vi "SV Read All Data.vi"(7 "reader ID":string="AllData", 8 "error in (no error)":errorcluster, 11 "buffer":refnum<data-value>) -> (0 "error out":errorcluster, 2 "waveforms":waveform(dbl)[](array[waveform]), 3 "buffer out":refnum<data-value>)   [LabVIEW 2017]
doc: "Adds buffering to stimulus-response applications. You must manually select the polymorphic instance to use."
uses:
  <vilib>/addons/_NISVFA/_Shared subVIs/Data Objects/Waveforms (DBL)/Waveforms (N Ch).lvclass
  C:/Program Files (x86)/National Instruments/LabVIEW 2017/vi.lib/addons/_NISVFA/_Shared subVIs/Data Objects/Data/Data.lvclass
  <vilib>/addons/_NISVFA/_Shared subVIs/Data Objects/Data/Data.lvclass/Data.ctl
  <vilib>/addons/_NISVFA/_Shared subVIs/Data Objects/Waveforms (DBL)/Waveforms (N Ch).lvclass/Waveforms (N Ch).ctl
  <vilib>/addons/_NISVFA/_Shared subVIs/Data Objects/Waveforms (DBL)/Read Mode for Deleting Stale Data.vi
  <vilib>/addons/_NISVFA/_Shared subVIs/Data Objects/subVIs/Get Data Timestamp.vi
  <vilib>/addons/_NISVFA/_Shared subVIs/Common/sv_Convert Timestamp to Relative Index.vi
  <vilib>/addons/_NISVFA/_Shared subVIs/Data Objects/subVIs/Get Data Length.vi
  <vilib>/addons/_NISVFA/_Shared subVIs/Common/SV Get Data Subset.vi
  <vilib>/addons/_NISVFA/_Shared subVIs/Common/svc_Copy Waveform Subset (Index).vi
  <vilib>/addons/_NISVFA/_Shared subVIs/Common/sv_Get NI Property Name String.vi
  <vilib>/addons/_NISVFA/_Shared subVIs/Data Objects/subVIs/Get Oldest of ReaderTimestamps.vi
  <vilib>/addons/_NISVFA/_Shared subVIs/Data Objects/subVIs/Set Data Timestamp.vi
  <vilib>/addons/_NISVFA/_Shared subVIs/Data Objects/subVIs/Set Data Length.vi
  <vilib>/addons/_NISVFA/_Shared subVIs/Common/svc_Get Waveform Subset (Index).vi
  <vilib>/addons/_NISVFA/_Shared subVIs/Common/svc_Copy Array Subset (Index).vi
  <vilib>/addons/_NISVFA/_Shared subVIs/Common/svc_Get Array Subset (Index).vi
  <vilib>/addons/_NISVFA/_Shared subVIs/Common/svc_Coerce Index and Length.vi
  <vilib>/addons/_NISVFA/_Shared subVIs/Common/svc_Conditional Merge Error.vi
  <vilib>/Utility/error.llb/Trim Whitespace.vi
  <vilib>/addons/_NISVFA/_Shared subVIs/Data Objects/Data/Data.lvclass
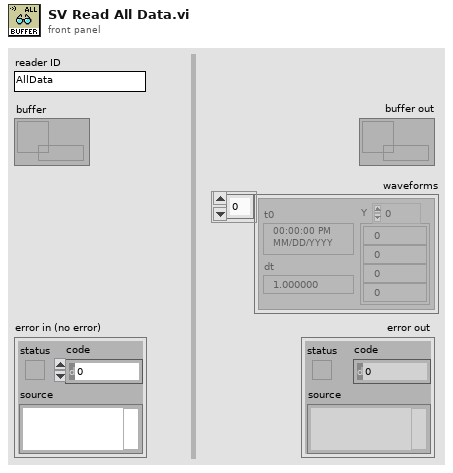
[diagram p1: front panel]
types:
  T1 = enum16{"Data Ready", "First Sample Not Yet Available", "Last Sample Not Yet Available", "Data No Longer Available"}
  T2 = typedef "svc_Delete Data Options (enum).ctl" = enum16{"Write", "Read", "Release"}
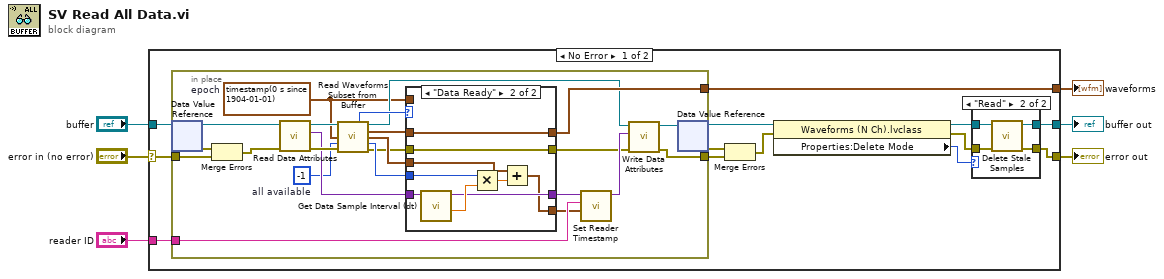
[diagram p0: block diagram]
diagram:
  n1 = case shown="No Error" "error in (no error)" {
    selector: "error in (no error)" -> [w16 w61]
    tunnel: "buffer" -> [w19 w62]
    tunnel: [w11 w62] -> w5
    tunnel: [w18 _] -> w4
    tunnel: [w8 w61] -> w3
    tunnel: "reader ID" -> [w17 _]
    frame No Error {
      n2 = in-place {
        in-place-border: [w31] -> w15
        in-place-border: [w44] -> w18
        in-place-border: w16 -> [w39]
        in-place-border: w17 -> [w29]
        w36 = -1  # all available
        w27 = timestamp(0 s since 1904-01-01)  # epoch
        n3 = in-place-dvr #1(w19) -> (w26:refnum<class "Waveforms (N Ch).lvclass">, w38:errorcluster)
        n4 = Merge Errors(w38, w39) -> (w37:errorcluster)
        n5 = call <vilib>:"Read Data Attributes.vi"("error in (no error)"=w37, "Data in"=w26) -> ("error out"=w41:errorcluster, "data attributes"=w40:variant, "Data out"=w46:refnum<class "Waveforms (N Ch).lvclass">)  [unwired: 7 in]
        n6 = call <vilib>:"Read Waveforms Subset from Buffer.vi"("Waveforms (N Ch)"=w46, "timestamp"=w27, "block length"=w36, "error in (no error)"=w41) -> ("subset status"=w42:T1, "Waveforms (N Ch)"=w34:refnum<class "Waveforms (N Ch).lvclass">, "waveforms subset"=w45:waveform(dbl)[], "actual timestamp"=w48:timestamp, "actual length"=w47:i32, "error out"=w43:errorcluster)  [unwired: 5 in, 1 out]
        n7 = case shown="\"Data Ready\"" w42 {
          tunnel: [w51 w54] -> w32
          tunnel: w48 -> [_ w55]
          tunnel: w47 -> [_ w60]
          tunnel: w40 -> [w50 w57]
          tunnel: w45 -> [_ w56]
          tunnel: [_ w56] -> w44
          tunnel: w43 -> [w51 w54]
          tunnel: [w50 w53] -> w30
          tunnel: [w49 w52] -> w28
          tunnel: w27 -> [w49 _]
          frame Default {
          }
          frame "Data Ready" {
            n8 = call <vilib>:"Get Data Sample Interval (dt).vi"("variant in"=w57) -> ("dt [s]"=w58:dbl, "variant out"=w53:variant)  [unwired: 9 in]
            n9 = Multiply(x=w60, y=w58) -> (x*y=w59:dbl)
            n10 = Add(x=w55, y=w59) -> (x+y=w52:timestamp)
          }
        }
        n11 = call <vilib>:"Set Reader Timestamp.vi"("timestamp"=w28, "ID"=w29, "data attributes in"=w30) -> ("data attributes out"=w35:variant)  [unwired: 8 in]
        n12 = call <vilib>:"Write Data Attributes.vi"("error in (no error)"=w32, "data attributes"=w35, "Data in"=w34) -> ("error out"=w31:errorcluster, "Data out"=w33:refnum<class "Waveforms (N Ch).lvclass">)  [unwired: 7 in]
        n13 = in-place-dvr #1(w33) -> (w7:refnum<data-value>, w14:errorcluster)
      }
      n14 = Merge Errors(w14, w15) -> (w13:errorcluster)
      n15 = property class="Waveforms (N Ch).lvclass"(reference=w7, error in=w13) -> (reference out=w10:refnum<data-value>, error out=w9:errorcluster, "Properties:Delete Mode"=w12:T2)
      n16 = case shown="\"Read\"" w12 {
        tunnel: [w21 w24] -> w11
        tunnel: w10 -> [w21 w25]
        tunnel: w9 -> [w20 w23]
        tunnel: [w20 w22] -> w8
        frame Default {
        }
        frame "Read" {
          n17 = call <vilib>:"Delete Stale Samples.vi"("error in (no error)"=w23, "buffer"=w25) -> ("error out"=w22:errorcluster, "buffer"=w24:refnum<data-value>)  [unwired: 6 in, 2 out]
        }
      }
    }
    frame Error {
    }
  }
  "buffer out" <- w5
  "error out" <- w3
  "waveforms" <- w4
